vi "load view plugin.vi"(11 "error in (no error)":errorcluster) -> (4 "view plugin":refnum<class "Abstract View.lvclass">, 15 "error out":errorcluster)   [LabVIEW 2022 SP3]
uses:
  Abstract View/Abstract View.lvlibp/Abstract View.lvclass
  <vilib>/Utility/error.llb/Error Cluster From Error Code.vi
  <vilib>/ErrorRing/Error Ring.xnode
  <vilib>/regexp/Match Regular Expression.xnode
  <vilib>/Utility/LVLibp/NI_PackedLibraryUtility.lvlib
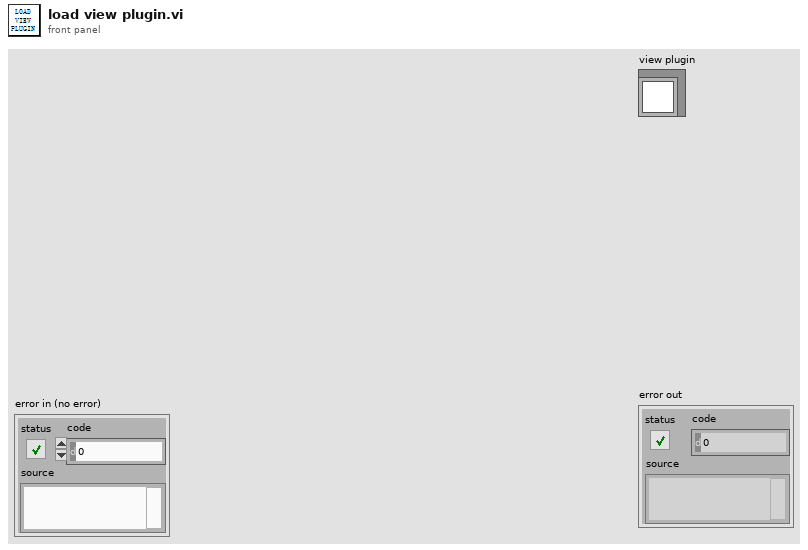
[diagram p1: front panel]
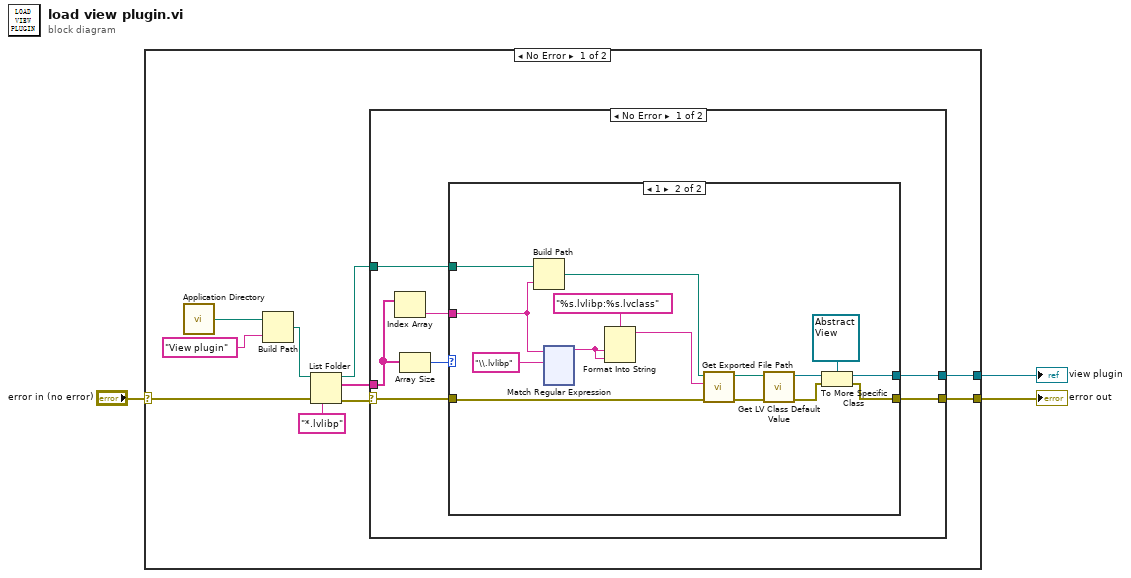
[diagram p0: block diagram]
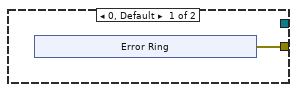
[diagram p2: hidden frame]
diagram:
  n1 = case shown="No Error" "error in (no error)" {
    selector: "error in (no error)" -> [w9 w160]
    tunnel: [w5 w160] -> w2
    tunnel: [w4 _] -> w1
    frame No Error {
      n2 = call <vilib>:"Application Directory.vi"() -> ("Application Directory"=w13:path)
      n3 = Build Path(base path=w13, name or relative path="View plugin") -> (appended path=w11:path)
      n4 = List Folder(path=w11, pattern="*.lvlibp", error in=w9) -> (path out=w6:path, filenames=w7:string[], error out=w8:errorcluster)  [unwired: 1 in, 1 out]
      n5 = case shown="No Error" w8 {
        selector: w8 -> [w16 w159]
        tunnel: w7 -> [w19 _]
        tunnel: w6 -> [w17 _]
        tunnel: [w15 w159] -> w5
        tunnel: [w14 _] -> w4
        frame No Error {
          n6 = Index Array(array=w19) -> (element=w18:string)  [unwired: 1 in]
          n7 = Array Size(array=w19) -> (size(s)=w20:i32)
          n8 = case shown="1" w20 {
            tunnel: w18 -> [_ w40]
            tunnel: w17 -> [_ w41]
            tunnel: w16 -> [_ w35]
            tunnel: [w21 w29] -> w15
            tunnel: [_ w28] -> w14
            frame 0, Default {
              n9 = xnode "Error Ring"() -> ("error out"=w21:errorcluster)
            }
            frame 1 {
              n10 = Build Path(base path=w41, name or relative path=w40) -> (appended path=w38:path)
              n11 = xnode "Match Regular Expression"("input string"=w40, "regular expression"="\\.lvlibp") -> ("before match"=w27:string)  [unwired: 4 in, 4 out]
              n12 = Format Into String(format string="%s.lvlibp:%s.lvclass", w27, w27) -> (resulting string=w36:string)  [unwired: 2 in, 1 out]
              n13 = call <vilib>:"Get Exported File Path.vi"("error in (no error)"=w35, "qualified name"=w36, "packed library path"=w38) -> ("error out"=w34:errorcluster, "path"=w33:path)  [unwired: 7 in]
              n14 = call <vilib>:"Get LV Class Default Value.vi"("error in (no error)"=w34, "class path"=w33) -> ("error out"=w30:errorcluster, "object"=w31:refnum<class>)  [unwired: 8 in]
              n15 = To More Specific Class(target class=refnum<class "Abstract View.lvclass"> refnum ("Abstract View.lvlibp:Abstract View.lvclass"), reference=w31, error in=w30) -> (specific class reference=w28:refnum<class "Abstract View.lvclass">, error out=w29:errorcluster)
            }
          }
        }
        frame Error {
        }
      }
    }
    frame Error {
    }
  }
  "error out" <- w2
  "view plugin" <- w1
